vi "SetTCGEnb.vi"(8 "错误输入（无错误）":errorcluster, 10 "TCG使能":i32) -> (0 "错误输出":errorcluster)   [LabVIEW 2014]
uses:
  ZXUTConfigMgr.dll
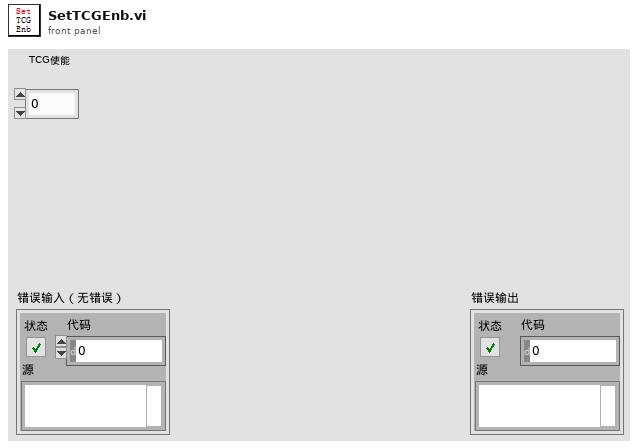
[diagram p1: front panel]
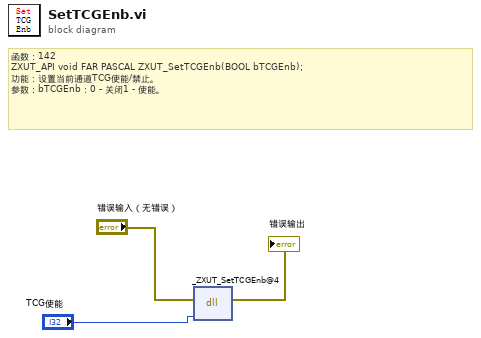
[diagram p0: block diagram]
diagram:
  # "函数：142\nZXUT_API void\tFAR PASCAL ZXUT_SetTCGEnb(BOOL bTCGEnb);\n功能：设置当前通道TCG使能/禁止。\n参数：bTCGEnb：0 - 关闭1 - 使能。"
  n1 = dll-call lib="PTH2eabs D软件超声实时监测软件ZXUTAppDemo(华南理工V02.00)X86DllZXUTConfigMgr.dll" fn="_ZXUT_SetTCGEnb@4"(error in="错误输入（无错误）", "bTCGEnb"="TCG使能") -> (error out=→"错误输出":errorcluster)  [unwired: 4 in, 1 out]
